vi "Test Cell Client.vi"() -> ()   [LabVIEW 2020]
uses:
  <vilib>/Skyline/Tag/Shared/typedefs/DataType.ctl
  <vilib>/Skyline/Tag/Wrapper/Wrapper_class/Read Tag (Boolean).vi
  <vilib>/Skyline/Message/HTTP Wrapper/NI Skyline Message HTTP.lvclass
  <vilib>/Skyline/Tag/Wrapper/Wrapper_class/NI Skyline Tag.lvclass
  <vilib>/Skyline/Tag/Shared/NI Skyline Tag.lvlib
  <vilib>/Skyline/Tag/Wrapper/Wrapper HTTP_class/NI Skyline Tag HTTP.lvclass
panel:
  in  "Send Log":bool
  out "Pressure":dbl[][](graph)
  out "Numeric":i32
  in  "Stop":bool
  in  "Refresh Button":bool
  in  "System":string(combo)="NI_cRIO-9049--SN-01234567--MAC-00-80-2F-AA-AA-AA"
  in  "Stop Test":bool
  out "Logging":bool
  in  "Start Test":bool
  out "Temperature":dbl[][](graph)
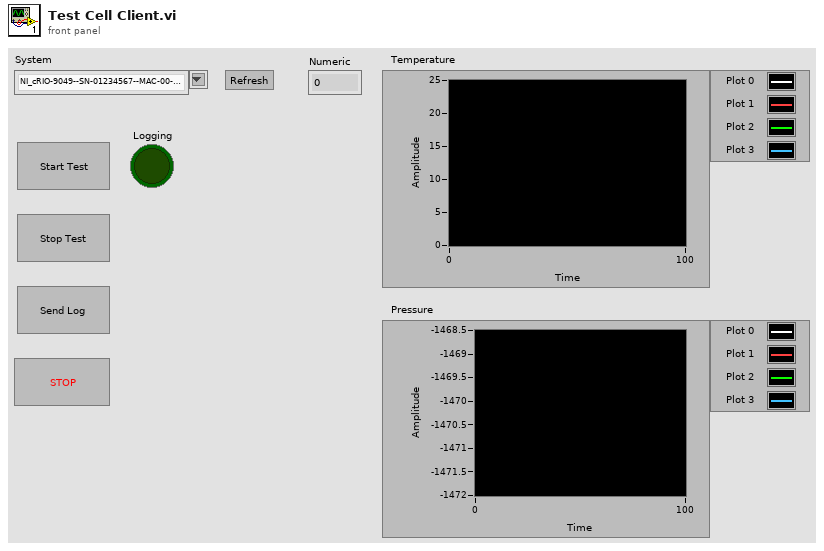
[diagram p1: front panel]
types:
  T1 = typedef "NI Skyline Tag.lvlib/DataType.ctl" = enum32{"Double", "I32", "String", "Boolean", "U64", "Timestamp"}
  T2 = typedef "NI Skyline Tag.lvlib/Tag Value Cluster.ctl" = cluster{"Path":string, "Workspace ID":string, "Data Type":T1, "Value":string, "Time Stamp":timestamp}
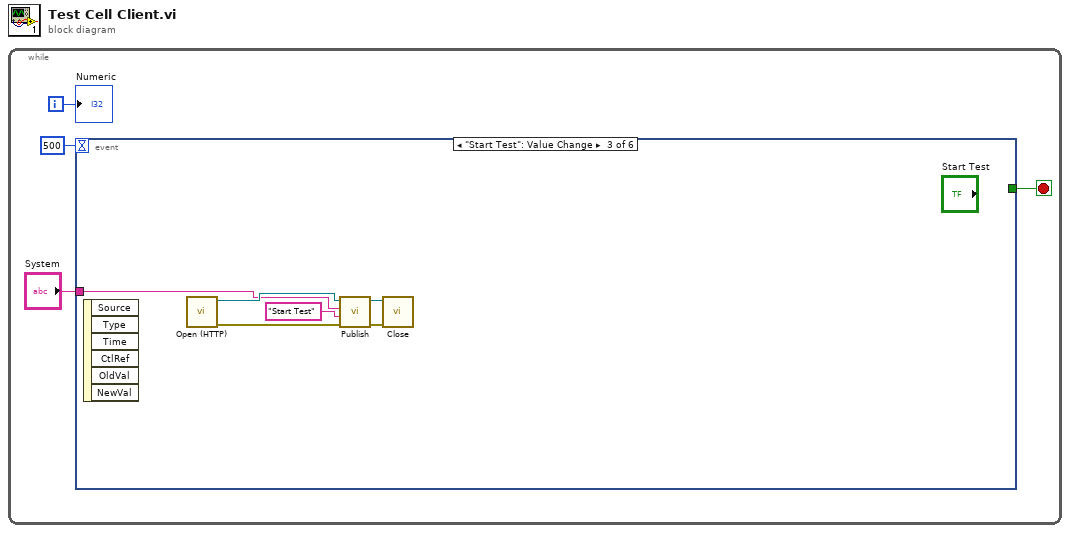
[diagram p0: block diagram]
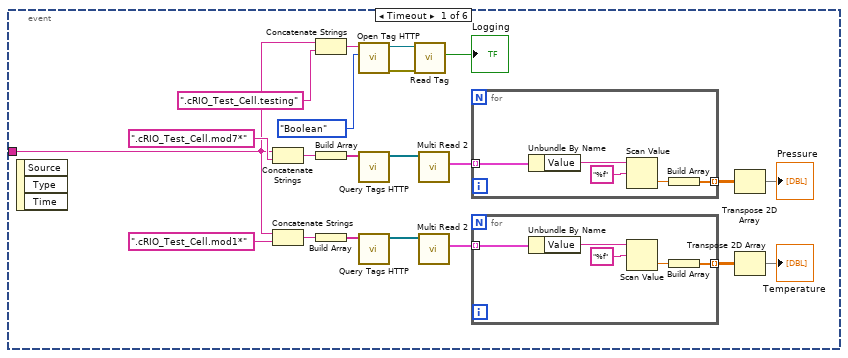
[diagram p2: hidden frame]
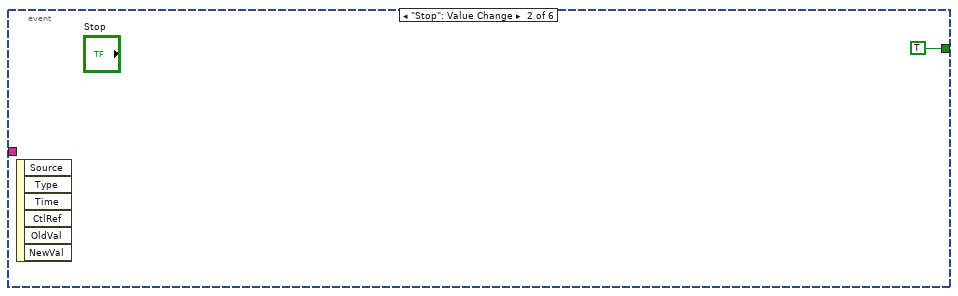
[diagram p3: hidden frame]
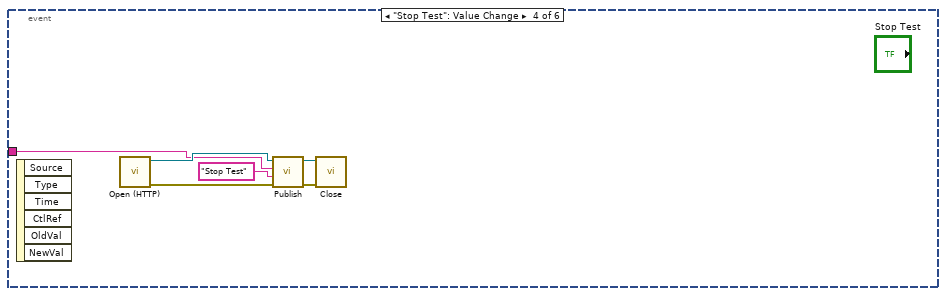
[diagram p4: hidden frame]
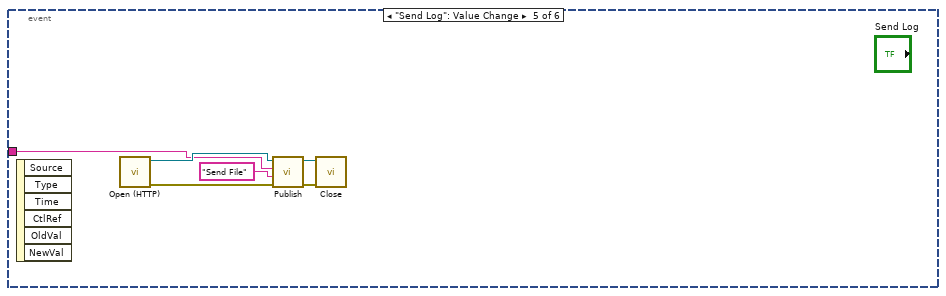
[diagram p5: hidden frame]
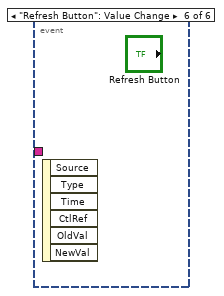
[diagram p6: hidden frame]
diagram:
  n1 = while {
    i -> [w2]
    stop <- w3 stop-if-true
    n2 = event shown="[2] \"Start Test\": Value Change" {
      selector: _ -> [_ _ _ _ _ _]
      dyn-events: _ -> [_ _ _ _ _ _]
      timeout: 500 -> [_ _ _ _ _ _]
      tunnel: "System" -> [w6 _ w38 w43 w49 _]
      tunnel: [_ TRUE _ _ _ _] -> w3
      event Timeout {
        n3 = event-data() -> ()  [unwired: 1 in, 3 out]
        n4 = Concatenate Strings(w6, ".cRIO_Test_Cell.mod7*" ("element")) -> (w15:string)
        n5 = Concatenate Strings(w6, ".cRIO_Test_Cell.mod1*" ("element")) -> (w22:string)
        n6 = Concatenate Strings(w6, ".cRIO_Test_Cell.testing" ("element")) -> (w8:string)
        n7 = Build Array(w15) -> (w16:string[])
        n8 = Build Array(w22) -> (w21:string[])
        n9 = call <vilib>:"Open Tag HTTP.vi"("Data Type"=DataType."Boolean" ("data type"), "path"=w8) -> ("error out"=w9:errorcluster, "tag"=w10:refnum<class "NI Skyline Tag.lvclass">)  [unwired: 8 in]
        n10 = call <vilib>:"Query Tags HTTP.vi"("paths"=w16) -> ("tags"=w13:refnum<class "NI Skyline Tag.lvclass">[])  [unwired: 8 in, 2 out]
        n11 = call <vilib>:"Query Tags HTTP.vi"("paths"=w21) -> ("tags"=w24:refnum<class "NI Skyline Tag.lvclass">[])  [unwired: 8 in, 2 out]
        n12 = call-poly <vilib>:"Read Tag.vi"("error in (no error)"=w9, "tag in"=w10) -> ("value"=→"Logging":bool)  [unwired: 5 in, 4 out]
        n13 = call <vilib>:"Multi Read 2.vi"("tags in"=w13) -> ("tag clusters"=w14:T2[])  [unwired: 8 in, 2 out]
        n14 = call <vilib>:"Multi Read 2.vi"("tags in"=w24) -> ("tag clusters"=w23:T2[])  [unwired: 8 in, 2 out]
        n15 = for {
          tunnel: w14 -> [w30] mode=indexing
          tunnel: [w26] -> w17 mode=indexing
          n16 = Unbundle By Name(w30) -> ("Value"=w29:string)
          n17 = Scan Value(string=w29, format string="%f") -> (value=w27:dbl)  [unwired: 1 in, 1 out]
          n18 = Build Array(w27) -> (w26:dbl[])
        }
        n19 = for {
          tunnel: w23 -> [w35] mode=indexing
          tunnel: [w31] -> w20 mode=indexing
          n20 = Unbundle By Name(w35) -> ("Value"=w34:string)
          n21 = Scan Value(string=w34, format string="%f") -> (value=w32:dbl)  [unwired: 1 in, 1 out]
          n22 = Build Array(w32) -> (w31:dbl[])
        }
        n23 = Transpose 2D Array(2D array=w17) -> (transposed array=→"Pressure":dbl[][])
        n24 = Transpose 2D Array(2D array=w20) -> (transposed array=→"Temperature":dbl[][])
      }
      event "Stop": Value Change {
        n25 = event-data() -> ()  [unwired: 1 in, 6 out]
      }
      event "Start Test": Value Change {
        n26 = event-data() -> ()  [unwired: 1 in, 6 out]
        n27 = call <vilib>:"Open (HTTP).vi"() -> ("error out"=w41:errorcluster, "message session"=w42:refnum<class "NI Skyline Message HTTP.lvclass">)  [unwired: 10 in]
        n28 = call-dynamic "Publish.vi"("error in (no error)"=w41, "message"="Start Test", "topic"=w38, "message session in"=w42) -> ("error out"=w39:errorcluster, "message session out"=w40:refnum<class "NI Skyline Message HTTP.lvclass">)  [unwired: 6 in]
        n29 = call-dynamic "Close.vi"("error in (no error)"=w39, "message session"=w40) -> ()  [unwired: 9 in, 1 out]
      }
      event "Stop Test": Value Change {
        n30 = event-data() -> ()  [unwired: 1 in, 6 out]
        n31 = call <vilib>:"Open (HTTP).vi"() -> ("error out"=w47:errorcluster, "message session"=w48:refnum<class "NI Skyline Message HTTP.lvclass">)  [unwired: 10 in]
        n32 = call-dynamic "Publish.vi"("error in (no error)"=w47, "message"="Stop Test", "topic"=w43, "message session in"=w48) -> ("error out"=w45:errorcluster, "message session out"=w46:refnum<class "NI Skyline Message HTTP.lvclass">)  [unwired: 6 in]
        n33 = call-dynamic "Close.vi"("error in (no error)"=w45, "message session"=w46) -> ()  [unwired: 9 in, 1 out]
      }
      event "Send Log": Value Change {
        n34 = event-data() -> ()  [unwired: 1 in, 6 out]
        n35 = call <vilib>:"Open (HTTP).vi"() -> ("error out"=w53:errorcluster, "message session"=w54:refnum<class "NI Skyline Message HTTP.lvclass">)  [unwired: 10 in]
        n36 = call-dynamic "Publish.vi"("error in (no error)"=w53, "message"="Send File", "topic"=w49, "message session in"=w54) -> ("error out"=w51:errorcluster, "message session out"=w52:refnum<class "NI Skyline Message HTTP.lvclass">)  [unwired: 6 in]
        n37 = call-dynamic "Close.vi"("error in (no error)"=w51, "message session"=w52) -> ()  [unwired: 9 in, 1 out]
      }
      event "Refresh Button": Value Change {
        n38 = event-data() -> ()  [unwired: 1 in, 6 out]
      }
    }
    "Numeric" <- w2
  }
